vi "example_read.vi"(6 "dvr":refnum<data-value>, 8 "error in (no error)":errorcluster, 10 "length":i32=-1, 11 "index in":i32=-1) -> (0 "error out":errorcluster, 1 "index":i32, 2 "y_axis":dbl[][](array[numeric]), 3 "x_axis":dbl[](array[numeric]))   [LabVIEW 2015, in "lv-graph.lvlib"]
uses:
  lv-graph.lvlib
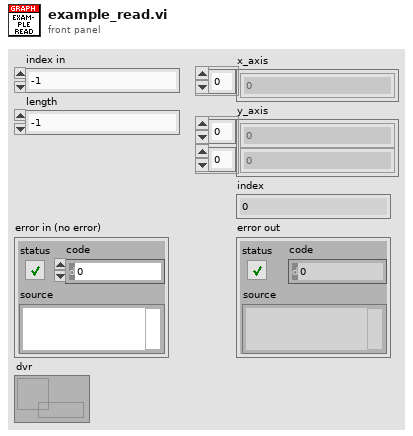
[diagram p1: front panel]
types:
  T1 = cluster{"index":i32, "x_axis":dbl[], "y_axis":dbl[][]}
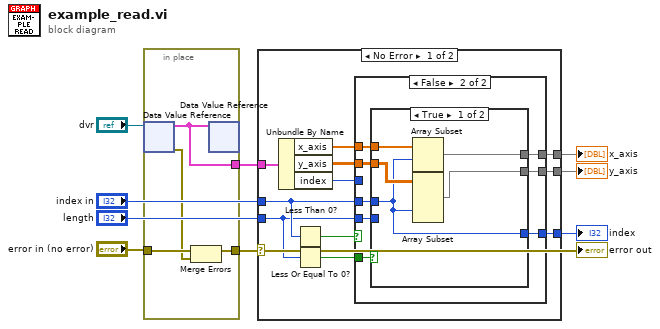
[diagram p0: block diagram]
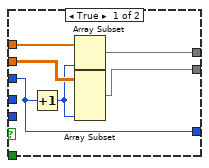
[diagram p2: hidden frame]
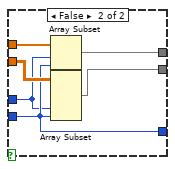
[diagram p3: hidden frame]
diagram:
  n1 = in-place {
    in-place-border: [w13] -> w2
    in-place-border: "error in (no error)" -> [w12]
    in-place-border: [w10] -> w6
    n2 = in-place-dvr #1("dvr") -> (w13:T1, w11:errorcluster)
    n3 = Merge Errors(w12, w11) -> (w10:errorcluster)
    n4 = in-place-dvr #1(w13) -> ()  [unwired: 2 out]
  }
  "error out" <- w6
  n5 = case shown="No Error" w6 {
    tunnel: w2 -> [w19 _]
    tunnel: "index in" -> [w18 _]
    tunnel: "length" -> [w17 _]
    tunnel: [w16 _] -> w3
    tunnel: [w15 _] -> w4
    tunnel: [w14 _] -> w5
    frame No Error {
      n6 = Unbundle By Name(w19) -> ("x_axis"=w20:dbl[], "y_axis"=w21:dbl[][], "index"=w24:i32)
      n7 = Less Than 0?(x=w18) -> (x < 0?=w22:bool)
      n8 = Less Or Equal To 0?(x=w17) -> (x <= 0?=w23:bool)
      n9 = case shown="False" w22 {
        tunnel: w20 -> [w30 w38]
        tunnel: w21 -> [w29 w37]
        tunnel: [w28 w36] -> w16
        tunnel: [w27 w35] -> w15
        tunnel: w24 -> [w26 _]
        tunnel: w18 -> [_ w34]
        tunnel: w17 -> [_ w32]
        tunnel: w23 -> [_ w33]
        tunnel: [w26 w31] -> w14
        frame True {
          n10 = Increment(x=w26) -> (x+1=w25:i32)
          n11 = Array Subset(array=w30, length=w25) -> (w28:dbl[])  [unwired: 1 in]
          n12 = Array Subset(array=w29, length (col)=w25) -> (w27:dbl[][])  [unwired: 3 in]
        }
        frame False {
          n13 = case shown="True" w33 {
            tunnel: w38 -> [w43 w49]
            tunnel: w37 -> [w42 w48]
            tunnel: [w41 w47] -> w36
            tunnel: [w40 w46] -> w35
            tunnel: w34 -> [w39 w44]
            tunnel: w32 -> [_ w45]
            tunnel: [w39 w45] -> w31
            frame True {
              n14 = Array Subset(array=w43, index=w39) -> (w41:dbl[])  [unwired: 1 in]
              n15 = Array Subset(array=w42, index (col)=w39) -> (w40:dbl[][])  [unwired: 3 in]
            }
            frame False {
              n16 = Array Subset(array=w49, index=w44, length=w45) -> (w47:dbl[])
              n17 = Array Subset(array=w48, index (col)=w44, length (col)=w45) -> (w46:dbl[][])  [unwired: 2 in]
            }
          }
        }
      }
    }
    frame Error {
    }
  }
  "index" <- w5
  "y_axis" <- w4
  "x_axis" <- w3
